vi "ConnectDataEntry.vi"(4 "MQTT Connect Data in":T4={"ClientID"="44be5e2ab7441ebaed34d7fa45d5e0", "Broker"={"address"="mqtt.thingspeak.com", "port"=1883, "connTimeout"=2000, "writeTimeout"=2000, "readTimeout"=2000, "subTimeout"=30000}, "Flags"={"reserved"=FALSE, "clean session"=TRUE, "will flag"=FALSE, "willQOS"=enum."At most once", "will retain"=FALSE, "password"=TRUE, "user name"=TRUE}, "User Info"={"User Name"="rgoetting", "Password"="2V41PDRHCBV3T4MR"}}) -> (1 "MQTT Connect Data out":T4={"ClientID"="44be5e2ab7441ebaed34d7fa45d5e0", "Broker"={"address"="mqtt.thingspeak.com", "port"=1883, "connTimeout"=2000, "writeTimeout"=2000, "readTimeout"=2000, "subTimeout"=30000}, "Flags"={"reserved"=FALSE, "clean session"=TRUE, "will flag"=FALSE, "willQOS"=enum."At most once", "will retain"=FALSE, "password"=TRUE, "user name"=TRUE}, "User Info"={"User Name"="rgoetting", "Password"="2V41PDRHCBV3T4MR"}})   [LabVIEW 2018]
uses:
  class/mqtt/mqttTypedef/mqttBroker.ctl
  class/mqtt/mqttTypedef/mqttConnectionFlags.ctl
  class/mqtt/mqttTypedef/mqttWillInformation.ctl
  <vilib>/Platform/TimedLoop/XDataNode/timing_clust.ctl
  <vilib>/Platform/TimedLoop/XDataNode/nitl_modes.ctl
  <vilib>/Platform/TimedLoop/XDataNode/wakeup.ctl
  <vilib>/platform/TimedLoop/XDataNode/XDataNode.xnode
  <vilib>/Platform/TimedLoop/XDataNode/XDNodeRunTimeDep.lvlib
panel:
  in  "MQTT Connect Data":T4={"ClientID"="44be5e2ab7441ebaed34d7fa45d5e0", "Broker"={"address"="mqtt.thingspeak.com", "port"=1883, "connTimeout"=2000, "writeTimeout"=2000, "readTimeout"=2000, "subTimeout"=30000}, "Flags"={"reserved"=FALSE, "clean session"=TRUE, "will flag"=FALSE, "willQOS"=enum."At most once", "will retain"=FALSE, "password"=TRUE, "user name"=TRUE}, "User Info"={"User Name"="rgoetting", "Password"="2V41PDRHCBV3T4MR"}}
  in  "Cancel":bool
  in  "ok":bool
  # "ThingSpeak Connection Data"
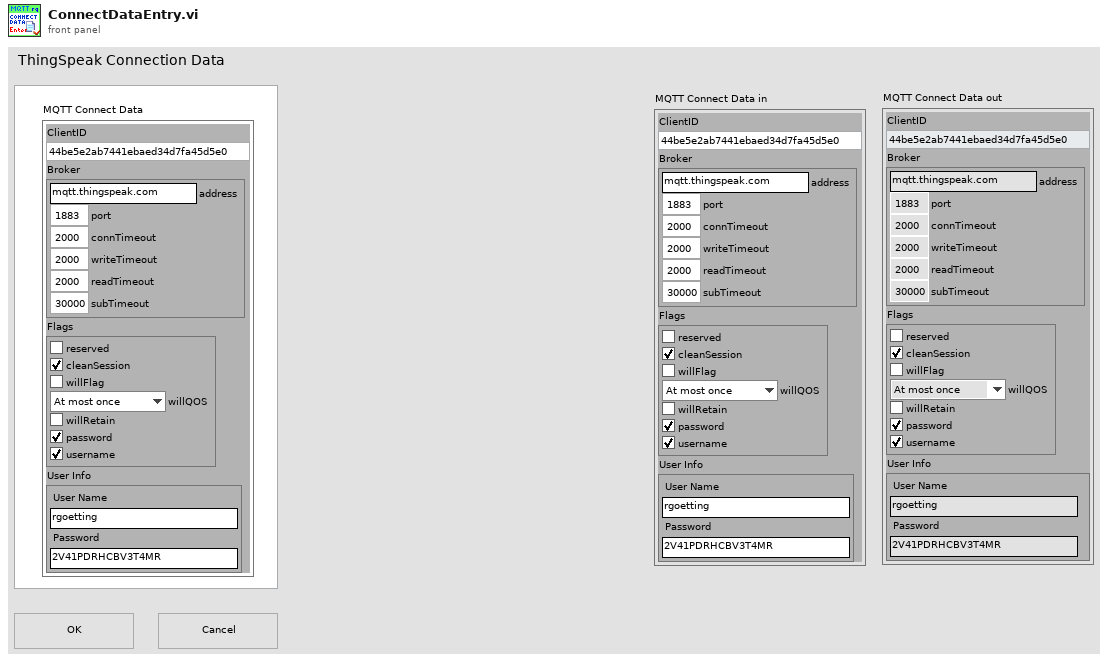
[diagram p1: front panel]
types:
  T1 = typedef "mqttBroker.ctl" = cluster{"address":string, "port":u16, "connTimeout":i32, "writeTimeout":i32, "readTimeout":i32, "subTimeout":i32}
  T2 = typedef "mqttConnectionFlags.ctl" = cluster{"reserved":bool, "clean session":bool, "will flag":bool, "willQOS":enum8{"At most once", "At least once", "Exactly once", "Reserved"}, "will retain":bool, "password":bool, "user name":bool}
  T3 = typedef "mqttWillInformation.ctl" = cluster{"User Name":string, "Password":string}
  T4 = cluster{"ClientID":string, "Broker":T1, "Flags":T2, "User Info":T3}
  T5 = typedef "XDNodeRunTimeDep.lvlib/timing_clust.ctl" = cluster{"Expected End [f-1]":u64, "Actual End [f-1]":u64, "Finished Late? [f-1]":bool, "Expected End [i-1]":u64, "Actual End [i-1]":u64, "Finished Late? [i-1]":bool, "Expected Start [i]":u64, "Actual Start [i]":u64, "Expected Start [f]":u64, "Actual Start [f]":u64, "Source Name":string, "Structure Name":string, "Period":i64, "Deadline":i64, "Offset":i64, "Start":i64, "Priority":i32, "Timeout":i32, "Mode":T6, "Wakeup Reason":T7, "Error":errorcluster, "Source Type":string, "Secondary Source Type":string, "Global End Time":u64, "Global Start Time":u64, "Frame Duration":u64, "Iteration Duration":u64, "Assigned CPU":i32, "I/O Scan Engine Mode":u32}
  T6 = typedef "XDNodeRunTimeDep.lvlib/nitl_modes.ctl" = enum32{"No Change", "Process missed periods, maintain original phase", "Discard missed periods, maintain original phase", "Process missed periods, ignore original phase", "Discard missed periods, ignore original phase"}
  T7 = typedef "XDNodeRunTimeDep.lvlib/wakeup.ctl" = enum32{"Normal", "Aborted", "Asynchronous wakeup", "Timing source error", "Timed loop error", "Timeout"}
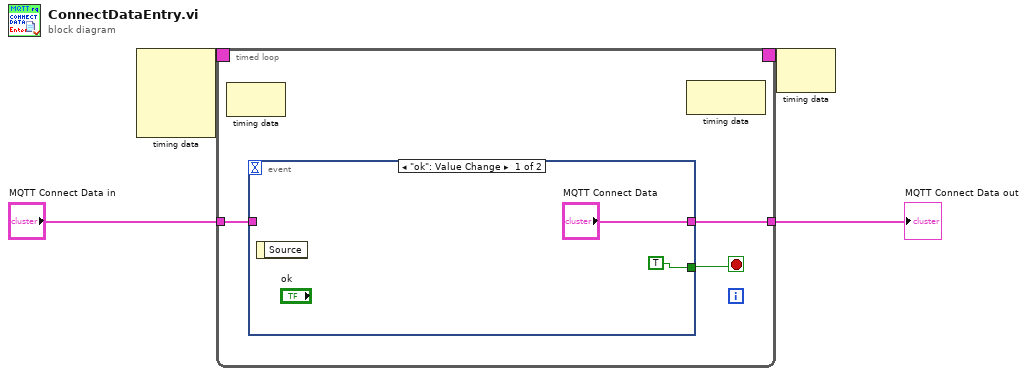
[diagram p0: block diagram]
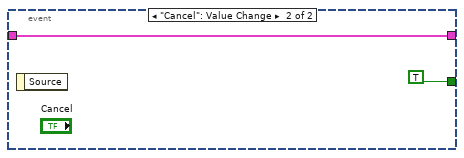
[diagram p2: hidden frame]
diagram:
  n1 = node-c288() -> (w4:T5)  [unwired: 4 in]
  n2 = timed-loop {
    timing: w4 -> [_]
    timing-out: [_] -> w3
    tunnel: "MQTT Connect Data in" -> [w6]
    tunnel: [w5] -> w1
    stop <- w7 stop-if-true
    n3 = node-c288() -> ()  [unwired: 1 in, 1 out]
    n4 = event shown="[0] \"ok\": Value Change" {
      selector: _ -> [_ _]
      dyn-events: _ -> [_ _]
      timeout: _ -> [_ _]
      tunnel: [TRUE ("NewVal") TRUE ("NewVal")] -> w7
      tunnel: w6 -> [_ w11]
      tunnel: ["MQTT Connect Data" w11] -> w5
      event "ok": Value Change {
        n5 = event-data() -> ()  [unwired: 1 in, 1 out]
      }
      event "Cancel": Value Change {
        n6 = event-data() -> ()  [unwired: 1 in, 1 out]
      }
    }
    n7 = node-c288() -> ()  [unwired: 1 in, 1 out]
  }
  "MQTT Connect Data out" <- w1
  n8 = node-c288(w3) -> ()  [unwired: 1 out]
